vi "Resonance_Test.vi"(0 "Semiconductor Module Context":T7, 1 "Pins Force":T4[](array[typedef]), 2 "Pins Meas":T4[](array[typedef]), 4 "FGEN_Parameters":T5[](array[typedef]) {"Trigger Mode" items=["Single", "Continuous", "Stepped", "Burst"]}, 5 "SCOPE_Parameters":T2[](array[typedef]) {"maximum input frequency" format="%.2f"; "input impedance" items=["1 mega ohm"=0, "50 ohms"=2]; "vertical offset" format="%.4f"; "vertical range" format="%.2f"; "vertical coupling" items=["AC", "DC", "Ground"]; "reference position" format="%#_13g"; "min sample rate" format="%^.2e"}, 6 "Published Data Id":T1, 7 "Source Type":enum16{"Static", "Dynamic"}(ring)) -> (19 "error out":errorcluster)   [LabVIEW 2023, in "Resonance.lvlib"]
doc: "Configures SMU/AWG and start generating; if using SMU it also measures back the voltage applied.\nThe SCOPE acquires N channels and averages the samples of each channel.\nThe Offset is computed by dividing the average value with the applied voltage or Vrms of Sine wave when using AWG"
uses:
  Resonance.lvlib
  ResourceHandling/ResourceHandling.lvlib
  <vilib>/NI_TestStand_SemiconductorModule/NI_TestStand_Semiconductor_Module.lvlibp
  <instrlib>/niScope/Controls/niScope trigger source digital.ctl
  <instrlib>/niFgen/niFgen.llb/niFgen_ctl Exported Signal Desination Values (ComboBox).ctl
  <vilib>/NI_TestStand_SemiconductorModule/NI_TestStand_Semiconductor_Module.lvlibp/PinMap/FGEN/PinsToNIFGenSessions.vi
  <vilib>/NI_TestStand_SemiconductorModule/NI_TestStand_Semiconductor_Module.lvlibp/PinMap/Scope/PinsToNISCOPESessions.vi
  <instrlib>/niScope/Acquire/Fetch/niScope Multi Fetch WDT.vi
  <vilib>/NI_TestStand_SemiconductorModule/NI_TestStand_Semiconductor_Module.lvlibp/PinMap/General/Publish/PublishDataPerSiteDoubleScalar.vi
  <vilib>/NI_TestStand_SemiconductorModule/NI_TestStand_Semiconductor_Module.lvlibp/PinMap/General/SemiconductorModuleContext.ctl
  <vilib>/NI_TestStand_SemiconductorModule/NI_TestStand_Semiconductor_Module.lvlibp/PinMap/TagProvider/TSM_Pin.ctl
  <instrlib>/niFgen/niFgen.llb/niFgen Trigger Mode.ctl
  ResourceHandling/TypeDefs/RH_FGEN_Parameters.ctl
  <instrlib>/niScope/Controls/niScope vertical coupling.ctl
  ResourceHandling/TypeDefs/RH_SCOPE_Parameters.ctl
  <vilib>/NI_TestStand_SemiconductorModule/NI_TestStand_Semiconductor_Module.lvlibp/PinMap/TagProvider/TSM_PublishedDataId.ctl
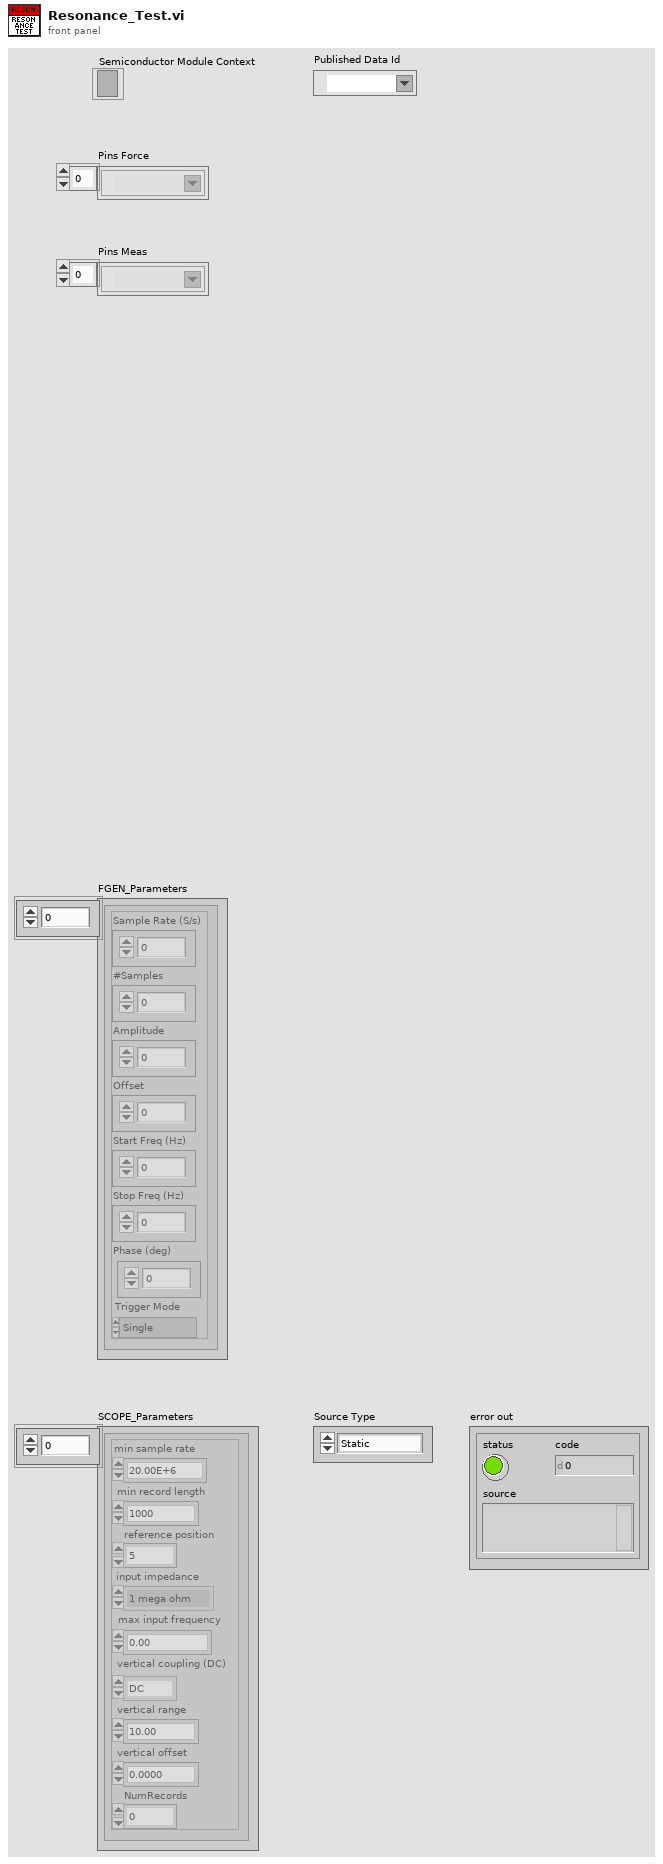
[diagram p1: front panel]
types:
  T1 = typedef "NI_TestStand_Semiconductor_Module.lvlibp/TSM_PublishedDataId.ctl" = tag
  T2 = typedef "ResourceHandling.lvlib/RH_SCOPE_Parameters.ctl" = cluster{"min sample rate":dbl, "min record length":i32, "reference position":dbl, "input impedance":u32, "maximum input frequency":dbl, "vertical coupling":T3, "vertical range":dbl, "vertical offset":dbl, "NumRecords":i32}
  T3 = typedef "niScope vertical coupling.ctl" = i32
  T4 = typedef "NI_TestStand_Semiconductor_Module.lvlibp/TSM_Pin.ctl" = tag
  T5 = typedef "ResourceHandling.lvlib/RH_FGEN_Parameters.ctl" = cluster{"Sample Rate (S/s)":dbl, "#Samples":i32, "Amplitude":dbl, "Offset":dbl, "Start Freq (Hz)":dbl, "Stop Freq (Hz)":dbl, "Phase (deg)":dbl, "Trigger Mode":T6}
  T6 = typedef "niFgen Trigger Mode.ctl" = i32
  T7 = typedef "NI_TestStand_Semiconductor_Module.lvlibp/SemiconductorModuleContext.ctl" = refnum<k7>
  T8 = typedef "niScope trigger source digital.ctl" = string
  T9 = typedef "niFgen_ctl Exported Signal Desination Values (ComboBox).ctl" = string
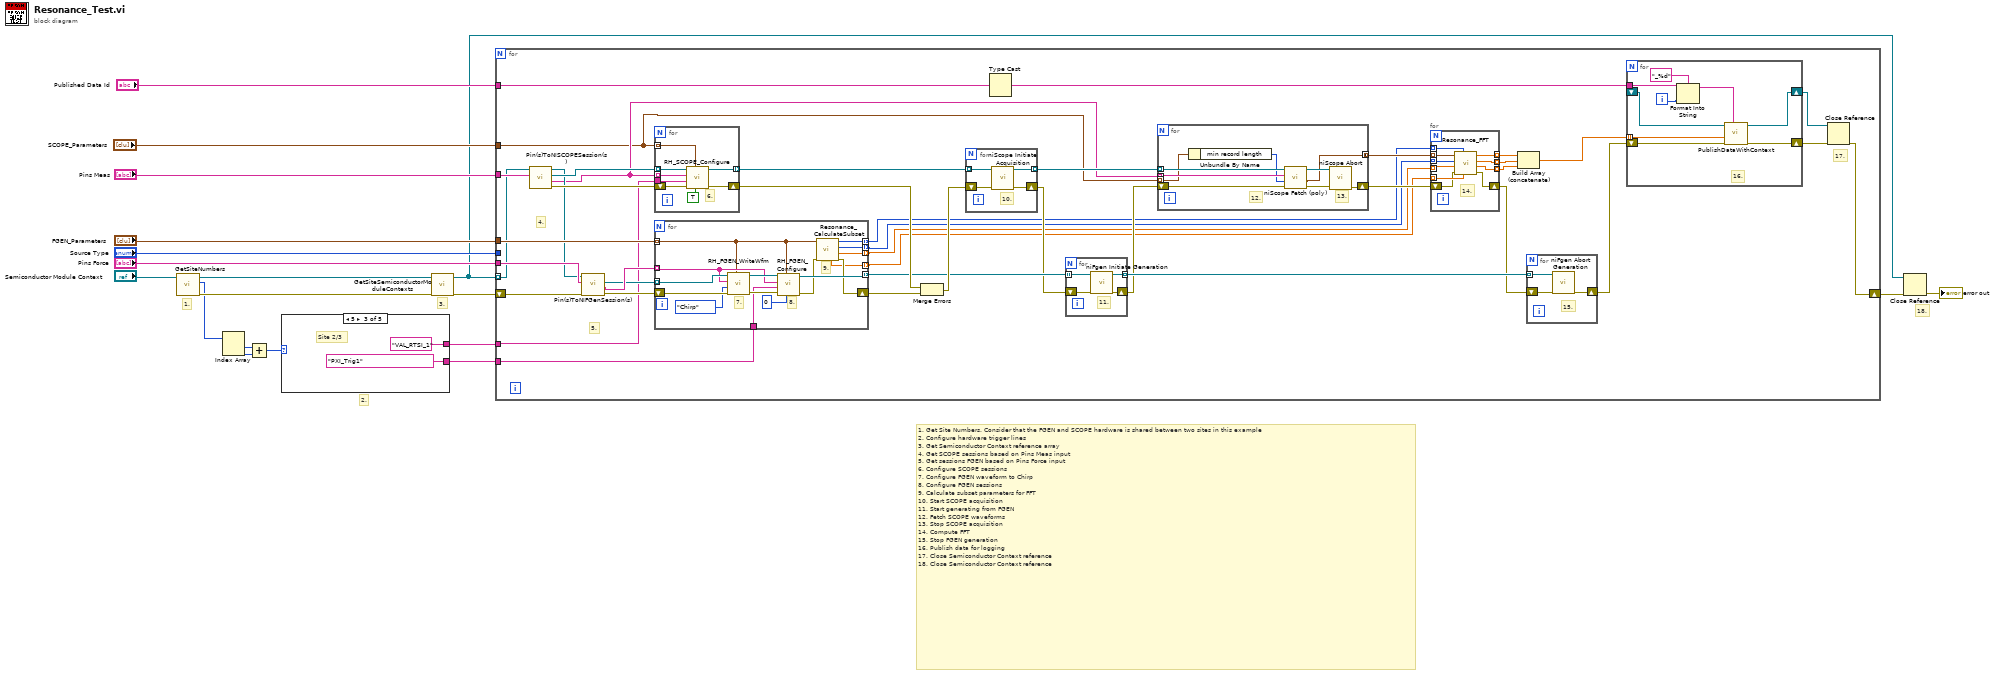
[diagram p0: block diagram]
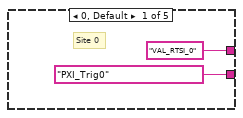
[diagram p2: hidden frame]
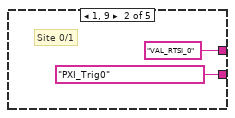
[diagram p3: hidden frame]
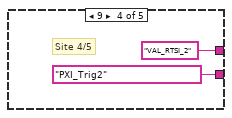
[diagram p4: hidden frame]
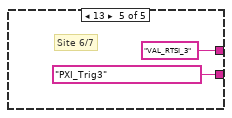
[diagram p5: hidden frame]
diagram:
  # "18."
  # "1. Get Site Numbers. Consider that the FGEN and SCOPE hardware is shared between two sites in this example\n2. Configure hardware trigger lines \n3. Get Semiconductor Context reference array\n4. Get SCOPE sessions based on Pins Meas input\n5. Get sessions FGEN based on Pins Force input\n6. Configure SCOPE sessions\n7. Configure FGEN waveform to Chirp\n8. Configure FGEN sessions\n9. Calculate subset parameters for FFT\n10. Start SCOPE acquisition\n11. Start generating from FGEN\n12. Fetch SCOPE waveforms\n13. Stop SCOPE acquisition\n14. Compute FFT\n15. Stop FGEN generation\n16. Publish data for logging\n17. Close Semiconductor Context reference\n18. Close Semiconductor Context reference"
  # "3."
  # "2."
  # "1."
  n1 = call <vilib>:"GetSiteNumbers.vi"("Semiconductor Module Context"="Semiconductor Module Context") -> ("error out"=w7:errorcluster, "Site Numbers"=w6:i32[], "Semiconductor Module Context Out"=w8:T7)  [unwired: 7 in, 1 out]
  n2 = Index Array(array=w6) -> (element #1=w5:i32, element #2=w4:i32)  [unwired: 2 in]
  n3 = Add(x=w5, y=w4) -> (x+y=w3:i32)
  n4 = case shown="5" w3 {
    tunnel: [T9 "PXI_Trig0" ("Output Terminal (do not export)") T9 "PXI_Trig0" ("Output Terminal (do not export)") T9 "PXI_Trig1" ("Output Terminal (do not export)") T9 "PXI_Trig2" ("Output Terminal (do not export)") T9 "PXI_Trig3" ("Output Terminal (do not export)")] -> w2
    tunnel: [T8 "VAL_RTSI_0" ("trigger source") T8 "VAL_RTSI_0" ("trigger source") T8 "VAL_RTSI_1" ("trigger source") T8 "VAL_RTSI_2" ("trigger source") T8 "VAL_RTSI_3" ("trigger source")] -> w1
    frame 0, Default {
      # "Site 0"
    }
    frame 1, 9 {
      # "Site 0/1"
    }
    frame 5 {
      # "Site 2/3"
    }
    frame 9 {
      # "Site 4/5"
    }
    frame 13 {
      # "Site 6/7"
    }
  }
  n5 = call <vilib>:"GetSiteSemiconductorModuleContexts.vi"("error in (no error)"=w7, "Semiconductor Module Context"=w8) -> ("error out"=w19:errorcluster, "Site Semiconductor Module Contexts"=w11:T7[])  [unwired: 8 in]
  n6 = for {
    tunnel: w11 -> [w55] mode=indexing
    tunnel: "Source Type" -> [_]
    tunnel: "Pins Force" -> [w69]
    tunnel: "FGEN_Parameters" -> [w68]
    tunnel: "Pins Meas" -> [w67]
    tunnel: "SCOPE_Parameters" -> [w39]
    tunnel: "Published Data Id" -> [w62]
    shift-right: [w58] -> w12
    shift-left: w19 -> [w70]
    tunnel: w2 -> [w53]
    tunnel: w1 -> [w52]
    # "17."
    # "5."
    # "4."
    n7 = call-poly <vilib>:"Pin(s)ToNISCOPESession(s).vi"("Pins"=w67, "Semiconductor Module Context"=w55) -> ("error out"=w65:errorcluster, "Channel Lists"=w40:string[], "Instrument Sessions"=w66:refnum<k15>[], "Semiconductor Module Context Out"=w54:T7)  [unwired: 5 in, 1 out]
    n8 = call-poly <vilib>:"Pin(s)ToNIFGenSession(s).vi"("error in (no error)"=w70, "Pins"=w69, "Semiconductor Module Context"=w54) -> ("error out"=w57:errorcluster, "Channel Lists"=w64:string[], "Instrument Sessions"=w56:refnum<k15>[])  [unwired: 4 in, 2 out]
    n9 = for {
      tunnel: w56 -> [w85] mode=indexing
      tunnel: w64 -> [w81] mode=indexing
      tunnel: w68 -> [w77] mode=indexing
      tunnel: [w78] -> w47 mode=indexing
      shift-right: [w75] -> w51
      shift-left: w57 -> [w86]
      tunnel: w53 -> [w79]
      tunnel: [w74] -> w38 mode=indexing
      tunnel: [w73] -> w37 mode=indexing
      tunnel: [w72] -> w36 mode=indexing
      tunnel: [w71] -> w35 mode=indexing
      # "9."
      # "8."
      # "7."
      n10 = call "RH_FGEN_WriteWfm.vi"("FGEN Parameters"=w77, "error IO"=w86, "Wfm Type"=enum16{"Chirp", "MultiSine", "Sine"}."Chirp", "Channel Name"=w81, "FGEN Session In"=w85) -> ("error out"=w82:errorcluster, "FGEN Session Out"=w83:refnum<k15>)  [unwired: 5 in]
      n11 = call "RH_FGEN_Configure.vi"("Marker Position"=0, "FGEN Parameters"=w77, "error in"=w82, "Output Terminal (do not export)"=w79, "Channel Name"=w81, "FGEN Session In"=w83) -> ("error out"=w76:errorcluster, "FGEN Session Out"=w78:refnum<k15>)  [unwired: 4 in]
      n12 = call "Resonance_CalculateSubset.vi"("error in"=w76, "FGEN Parameters"=w77) -> ("error out"=w75:errorcluster, "dF"=w72:dbl, "Length"=w73:i32, "Index"=w74:i32, "Start Offset"=w71:dbl)  [unwired: 5 in]
    }
    n13 = for {
      tunnel: w66 -> [w93] mode=indexing
      tunnel: w40 -> [w91] mode=indexing
      shift-right: [w88] -> w50
      shift-left: w65 -> [w94]
      tunnel: w39 -> [w90] mode=indexing
      tunnel: w52 -> [w89]
      tunnel: [w87] -> w49 mode=indexing
      # "6."
      n14 = call "RH_SCOPE_Configure.vi"("Digital Trigger?"=TRUE, "SCOPE Global Parameters"=w90, "error in"=w94, "trigger source"=w89, "channels"=w91, "SCOPE Session In"=w93) -> ("error out"=w88:errorcluster, "SCOPE Session Out"=w87:refnum<k15>)  [unwired: 4 in]
    }
    n15 = Merge Errors(w50, w51) -> (w48:errorcluster)
    n16 = for {
      tunnel: w49 -> [w111] mode=indexing
      shift-right: [w109] -> w46
      shift-left: w48 -> [w110]
      tunnel: [w108] -> w44 mode=indexing
      # "10."
      n17 = call <instrlib>:"niScope Initiate Acquisition.vi"("instrument handle"=w111, "error in"=w110) -> ("instrument handle out"=w108:refnum<k15>, "error out"=w109:errorcluster)  [unwired: 12 in]
    }
    n18 = Type Cast(x=w62) -> (*(type *) &x=w61:string)  [unwired: 1 in]
    n19 = for {
      tunnel: w47 -> [w107] mode=indexing
      shift-right: [w105] -> w43
      shift-left: w46 -> [w106]
      tunnel: [w104] -> w45 mode=indexing
      # "11."
      n20 = call <instrlib>:"niFgen Initiate Generation.vi"("error in (no error)"=w106, "Instrument Handle"=w107) -> ("error out"=w105:errorcluster, "Instrument Handle Out"=w104:refnum<k15>)  [unwired: 8 in]
    }
    n21 = for {
      tunnel: w44 -> [w101] mode=indexing
      shift-right: [w99] -> w41
      shift-left: w43 -> [w100]
      tunnel: [w98] -> w42 mode=concatenating
      tunnel: w40 -> [w97] mode=indexing
      tunnel: w39 -> [w96] mode=indexing
      # "13."
      # "12."
      n22 = Unbundle By Name(w96) -> ("min record length"=w95:i32)
      n23 = call-poly <instrlib>:"niScope Fetch (poly).vi"("error in"=w100, "numSamples"=w95, "channels"=w97, "instrument handle"=w101) -> ("error out"=w102:errorcluster, "wfm"=w98:waveform(dbl)[], "instrument handle out"=w103:refnum<k15>)  [unwired: 4 in, 1 out]
      n24 = call <instrlib>:"niScope Abort.vi"("instrument handle"=w103, "error in"=w102) -> ("error out"=w99:errorcluster)  [unwired: 12 in, 1 out]
    }
    n25 = for {
      shift-right: [w115] -> w34
      shift-left: w41 -> [w116]
      tunnel: w42 -> [w121] mode=indexing
      tunnel: w36 -> [w118] mode=indexing
      tunnel: w35 -> [w117] mode=indexing
      tunnel: w38 -> [w120] mode=indexing
      tunnel: w37 -> [w119] mode=indexing
      tunnel: [w114] -> w32 mode=indexing
      tunnel: [w113] -> w31 mode=indexing
      tunnel: [w112] -> w30 mode=indexing
      # "14."
      n26 = call "Resonance_FFT.vi"("Start Offset"=w117, "Index"=w120, "error in"=w116, "dF"=w118, "Length"=w119, "Waveform"=w121) -> ("error out"=w115:errorcluster, "Phase"=w112:dbl, "Frequency"=w113:dbl, "Amplitude"=w114:dbl)  [unwired: 2 in]
    }
    n27 = Build Array (concatenate)(w32, w31, w30) -> (w33:dbl[])
    n28 = for {
      tunnel: w45 -> [w122] mode=indexing
      shift-right: [w124] -> w63
      shift-left: w34 -> [w123]
      # "15."
      n29 = call <instrlib>:"niFgen Abort Generation.vi"("error in (no error)"=w123, "Instrument Handle"=w122) -> ("error out"=w124:errorcluster)  [unwired: 8 in, 1 out]
    }
    n30 = for {
      tunnel: w61 -> [w130]
      shift-right: [w127] -> w60
      shift-left: w63 -> [w133]
      shift-right: [w126] -> w59
      shift-left: _ -> [w132]
      tunnel: w33 -> [w125] mode=indexing
      i -> [w129]
      # "16."
      n31 = Format Into String(format string="_%d", initial string=w130, w129) -> (resulting string=w128:string)  [unwired: 1 in, 1 out]
      n32 = call-poly <vilib>:"PublishDataWithContext.vi"("Published Data Id"=w128, "error in (no error)"=w133, "Data In"=w125, "Semiconductor Module Context"=w132) -> ("error out"=w127:errorcluster, "Semiconductor Module Context Out"=w126:T7)  [unwired: 6 in]
    }
    n33 = Close Reference(reference=w59, error in (no error)=w60) -> (error out=w58:errorcluster)
  }
  n34 = Close Reference(reference=w11, error in (no error)=w12) -> (error out=→"error out":errorcluster)
